vi "Fetch Min Max Waveform.vi"(8 "error in (no error)":errorcluster, 9 "Maximum Time (10000 ms)":u32=10000, 10 "Channel (1: Channel 1)":u16(ring)=1 items=["Channel 1"=1, "Channel 2"=2, "Channel 3"=3, "Channel 4"=4], 11 "VISA resource name":refnum<visa-resource-name>) -> (0 "error out":errorcluster, 1 "Max Waveform Data":waveform(dbl)(graph), 2 "Min Waveform Data":waveform(dbl)(graph), 3 "VISA resource name out":refnum<visa-resource-name>)   [LabVIEW 2011, in "Agilent DSO1000 Series.lvlib"]
doc: "Returns the min and maxwaveform the oscilloscope acquired for the specified channel. This VI only works in Peak Detect acquisiton mode.\n\nYou use the Initiate VI to start an acquisition on the channels that you enable with the Configure Channel VI. The oscilloscope acquires waveforms for the enabled channels concurrently. You must call this VI separately for each enabled channel to obtain the waveforms.\n\nYou can call the Read Waveform VI instead of using low-level VIs.\n\n<B>Note:</B> Use this VI only with other low-level VIs. The high-level VIs automatically incorporate this functionality. This VI does not check the instrument status."
uses:
  <instrlib>/Agilent DSO1000 Series/Agilent DSO1000 Series.lvlib
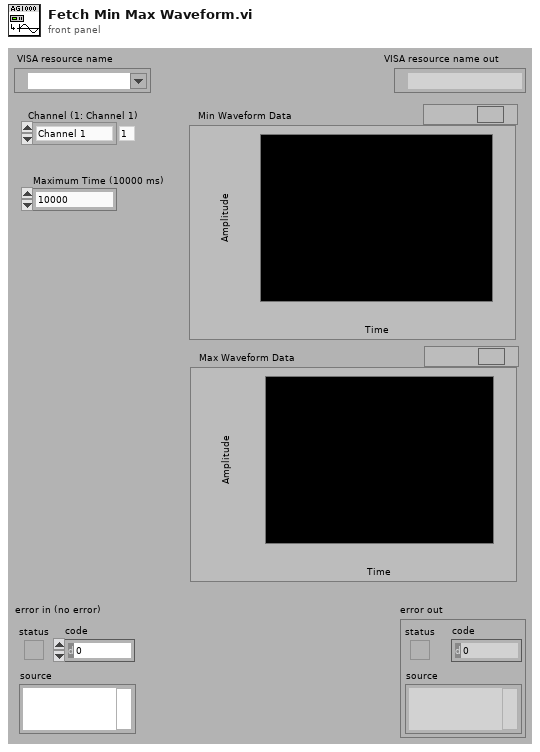
[diagram p1: front panel]
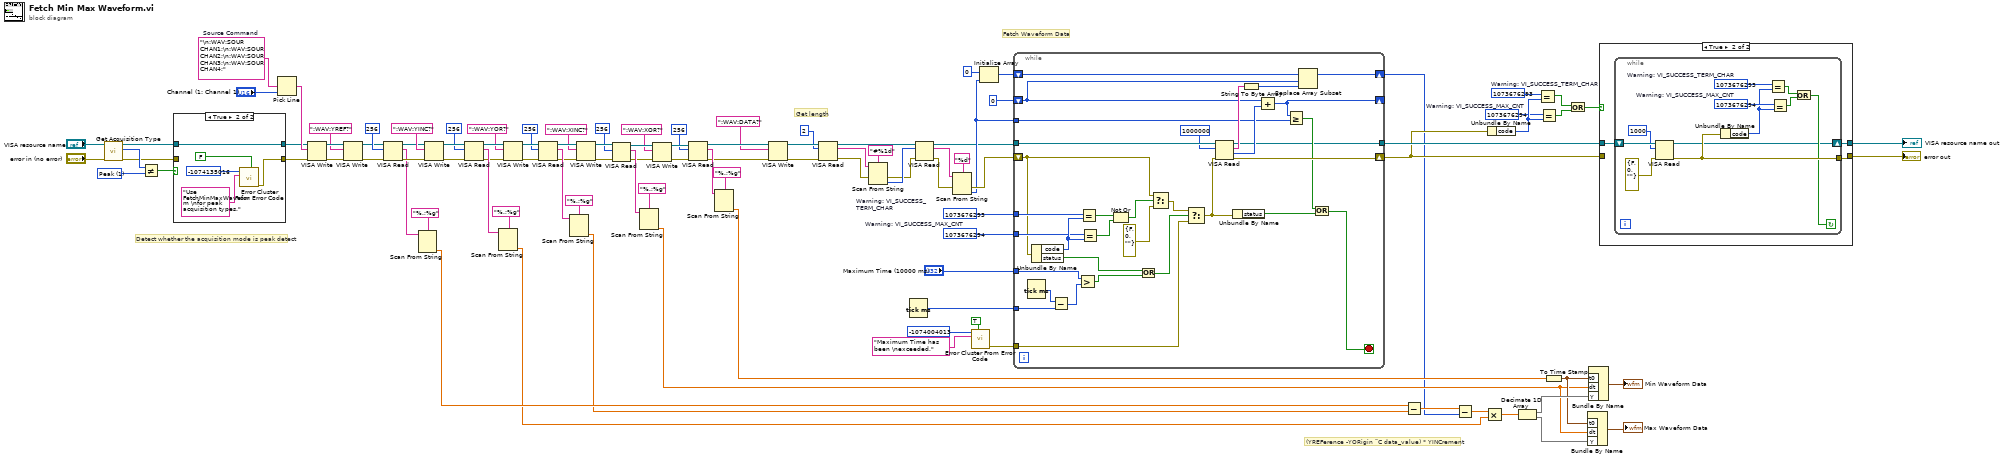
[diagram p0: block diagram]
diagram:
  w29 = 1 items=["Normal", "Peak", "Average"] ("y")
  w35 = 1073676294  # Warning: VI_SUCCESS_MAX_CNT
  w46 = 1073676293  # Warning: VI_SUCCESS_TERM_CHAR
  w51 = 1073676294  # Warning: VI_SUCCESS_MAX_CNT
  w52 = 1073676293  # Warning: VI_SUCCESS_TERM_CHAR
  w103 = "\n:WAV:SOUR CHAN1;\n:WAV:SOUR CHAN2;\n:WAV:SOUR CHAN3;\n:WAV:SOUR CHAN4;"  # Source Command
  # "(YREFerence -YORigin ¨C data_value) * YINCrement"
  # "Detect whether the acquisition mode is peak detect"
  # "Get length"
  # "Fetch Waveform Data"
  n1 = call <instrlib>:"Get Acquisition Type.vi"("error in (no error)"="error in (no error)", "VISA resource name"="VISA resource name") -> ("error out"=w25:errorcluster, "Acquisition Type"=w30:i32, "VISA resource name out"=w27:refnum<visa-resource-name>)  [unwired: 7 in]
  n2 = Not Equal?(x=w30, y=w29) -> (x != y?=w28:bool)
  n3 = case shown="True" w28 {
    tunnel: w27 -> [w107 w112]
    tunnel: [w107 w112] -> w26
    tunnel: w25 -> [w106 _]
    tunnel: [w106 w108] -> w24
    frame False {
    }
    frame True {
      n4 = call <vilib>:"Error Cluster From Error Code.vi"("is warning? (False)"=FALSE, "error message (\"\")"="Use FetchMinMaxWaveform \nfor peak  acquisition types.", "error code (0)"=-1074135016) -> ("error out"=w108:errorcluster)  [unwired: 6 in]
    }
  }
  n5 = Pick Line(multi-line string=w103, line index="Channel (1: Channel 1)") -> (output string=w104:string)  [unwired: 1 in]
  n6 = VISA Write(VISA resource name=w26, write buffer=w104, error in (no error)=w24) -> (VISA resource name out=w20:refnum<visa-resource-name>, error out=w19:errorcluster)  [unwired: 1 out]
  n7 = VISA Write(VISA resource name=w20, write buffer=":WAV:YREF?", error in (no error)=w19) -> (VISA resource name out=w21:refnum<visa-resource-name>, error out=w22:errorcluster)  [unwired: 1 out]
  n8 = VISA Read(VISA resource name=w21, byte count=u32 256, error in (no error)=w22) -> (VISA resource name out=w17:refnum<visa-resource-name>, read buffer=w14:string, error out=w16:errorcluster)  [unwired: 1 out]
  n9 = Scan From String(format string="%.;%g", input string=w14) -> (output 1=w13:dbl)  [unwired: 3 in, 3 out]
  n10 = VISA Write(VISA resource name=w17, write buffer=":WAV:YINC?", error in (no error)=w16) -> (VISA resource name out=w75:refnum<visa-resource-name>, error out=w74:errorcluster)  [unwired: 1 out]
  n11 = VISA Read(VISA resource name=w75, byte count=u32 256, error in (no error)=w74) -> (VISA resource name out=w100:refnum<visa-resource-name>, read buffer=w102:string, error out=w99:errorcluster)  [unwired: 1 out]
  n12 = Scan From String(format string="%.;%g", input string=w102) -> (output 1=w1:dbl)  [unwired: 3 in, 3 out]
  n13 = VISA Write(VISA resource name=w100, write buffer=":WAV:YOR?", error in (no error)=w99) -> (VISA resource name out=w97:refnum<visa-resource-name>, error out=w96:errorcluster)  [unwired: 1 out]
  n14 = VISA Read(VISA resource name=w97, byte count=u32 256, error in (no error)=w96) -> (VISA resource name out=w92:refnum<visa-resource-name>, read buffer=w94:string, error out=w91:errorcluster)  [unwired: 1 out]
  n15 = Scan From String(format string="%.;%g", input string=w94) -> (output 1=w2:dbl)  [unwired: 3 in, 3 out]
  n16 = VISA Write(VISA resource name=w92, write buffer=":WAV:XINC?", error in (no error)=w91) -> (VISA resource name out=w89:refnum<visa-resource-name>, error out=w88:errorcluster)  [unwired: 1 out]
  n17 = VISA Read(VISA resource name=w89, byte count=u32 256, error in (no error)=w88) -> (VISA resource name out=w84:refnum<visa-resource-name>, read buffer=w86:string, error out=w83:errorcluster)  [unwired: 1 out]
  n18 = Scan From String(format string="%.;%g", input string=w86) -> (output 1=w5:dbl)  [unwired: 3 in, 3 out]
  n19 = VISA Write(VISA resource name=w84, write buffer=":WAV:XOR?", error in (no error)=w83) -> (VISA resource name out=w81:refnum<visa-resource-name>, error out=w80:errorcluster)  [unwired: 1 out]
  n20 = VISA Read(VISA resource name=w81, byte count=u32 256, error in (no error)=w80) -> (VISA resource name out=w37:refnum<visa-resource-name>, read buffer=w78:string, error out=w36:errorcluster)  [unwired: 1 out]
  n21 = Scan From String(format string="%.;%g", input string=w78) -> (output 1=w72:dbl)  [unwired: 3 in, 3 out]
  n22 = VISA Write(VISA resource name=w37, write buffer=":WAV:DATA?" ("multi-line string"), error in (no error)=w36) -> (VISA resource name out=w71:refnum<visa-resource-name>, error out=w70:errorcluster)  [unwired: 1 out]
  n23 = VISA Read(VISA resource name=w71, byte count=u32 2, error in (no error)=w70) -> (VISA resource name out=w66:refnum<visa-resource-name>, read buffer=w67:string, error out=w68:errorcluster)  [unwired: 1 out]
  n24 = Scan From String(format string="#%1d", input string=w67, error in=w68) -> (error out=w63:errorcluster, output 1=w64:i32)  [unwired: 2 in, 2 out]
  n25 = Tick Count (ms)() -> (millisecond timer value=w53:u32)
  n26 = VISA Read(VISA resource name=w66, byte count=w64, error in (no error)=w63) -> (VISA resource name out=w54:refnum<visa-resource-name>, read buffer=w61:string, error out=w62:errorcluster)  [unwired: 1 out]
  n27 = Scan From String(format string="%d", input string=w61, error in=w62) -> (error out=w59:errorcluster, output 1=w55:i32)  [unwired: 2 in, 2 out]
  n28 = call <vilib>:"Error Cluster From Error Code.vi"("show call chain? (False)"=TRUE, "error message (\"\")"="Maximum Time has been \nexceeded." ("error message (\"\")"), "error code (0)"=-1074004013) -> ("error out"=w47:errorcluster)  [unwired: 6 in]
  n29 = Initialize Array(i8 0 ("element"), w55) -> (w57:i8[])
  n30 = while {
    shift-right: [w115] -> w3
    shift-left: w57 -> [w116]
    shift-right: [w123] -> _
    shift-left: 0 ("element") -> [w117]
    tunnel: w55 -> [w122]
    tunnel: w54 -> [w142]
    shift-right: [w126] -> w40
    shift-left: w59 -> [w136]
    tunnel: w53 -> [w145]
    tunnel: w52 -> [w140]
    tunnel: w51 -> [w139]
    tunnel: w47 -> [w129]
    tunnel: [w114] -> w41
    tunnel: "Maximum Time (10000 ms)" -> [w113]
    stop <- w119 stop-if-true
    n31 = Tick Count (ms)() -> (millisecond timer value=w144:u32)
    n32 = Unbundle By Name(w136) -> ("code"=w141:i32, "status"=w132:bool)
    n33 = Subtract(x=w144, y=w145) -> (x-y=w143:u32)
    n34 = Greater?(x=w113, y=w143) -> (0:w133:bool)
    n35 = Equal?(x=w140, y=w141) -> (x = y?=w138:bool)
    n36 = Equal?(x=w139, y=w141) -> (x = y?=w137:bool)
    n37 = Not Or(1:w137, 2:w138) -> (0:w135:bool)
    n38 = Or(x=w132, y=w133) -> (x .or. y?=w131:bool)
    n39 = Select(t=w136, s=w135, f=errorcluster {"status"=FALSE, "code"=0, "source"=""} ("error in (no error) 2")) -> (s? t:f=w130:errorcluster)
    n40 = Select(t=w130, s=w131, f=w129) -> (s? t:f=w128:errorcluster)
    n41 = VISA Read(VISA resource name=w142, byte count=u32 1000000, error in (no error)=w128) -> (VISA resource name out=w114:refnum<visa-resource-name>, read buffer=w125:string, return count=w124:u32, error out=w126:errorcluster)
    n42 = Unbundle By Name(w128) -> ("status"=w120:bool)
    n43 = String To Byte Array(string=w125) -> (unsigned byte array=w118:u8[])
    n44 = Add(x=w117, y=w124) -> (x+y=w123:u32)
    n45 = Greater Or Equal?(x=w123, y=w122) -> (x >= y?=w121:bool)
    n46 = Replace Array Subset(array=w116, new element=w118, index=w117) -> (w115:i8[])
    n47 = Or(x=w121, y=w120) -> (x .or. y?=w119:bool)
  }
  n48 = Subtract(x=w13, y=w2) -> (x-y=w12:dbl)
  n49 = Subtract(x=w12, y=w3) -> (x-y=w11:dbl[])
  n50 = Multiply(x=w11, y=w1) -> (x*y=w10:dbl[])
  n51 = Unbundle By Name(w40) -> ("code"=w45:i32)
  n52 = Decimate 1D Array(w10) -> (w8:dbl[], w7:dbl[])
  n53 = Equal?(x=w46, y=w45) -> (x = y?=w44:bool)
  n54 = Equal?(x=w35, y=w45) -> (x = y?=w43:bool)
  n55 = To Time Stamp(1:w72) -> (0:w6:timestamp)
  n56 = Or(x=w44, y=w43) -> (x .or. y?=w42:bool)
  n57 = Bundle By Name("t0"=w6, "dt"=w5, "Y"=w7) -> (→"Max Waveform Data":waveform(dbl))  [unwired: 1 in]
  n58 = Bundle By Name("t0"=w6, "dt"=w5, "Y"=w8) -> (→"Min Waveform Data":waveform(dbl))  [unwired: 1 in]
  n59 = case shown="True" w42 {
    tunnel: w41 -> [w147 w150]
    tunnel: w40 -> [w146 _]
    tunnel: [w147 w148] -> w39
    tunnel: [w146 w149] -> w38
    frame False {
    }
    frame True {
      n60 = while {
        shift-right: [w151] -> w148
        shift-left: w150 -> [w161]
        tunnel: [w154] -> w149
        stop <- w152 continue-if-true
        w157 = 1073676294  # Warning: VI_SUCCESS_MAX_CNT
        w158 = 1073676293  # Warning: VI_SUCCESS_TERM_CHAR
        n61 = VISA Read(VISA resource name=w161, byte count=u32 1000, error in (no error)=errorcluster {"status"=FALSE, "code"=0, "source"=""} ("error in (no error) 2")) -> (VISA resource name out=w151:refnum<visa-resource-name>, error out=w154:errorcluster)  [unwired: 2 out]
        n62 = Unbundle By Name(w154) -> ("code"=w153:i32)
        n63 = Equal?(x=w158, y=w153) -> (x = y?=w156:bool)
        n64 = Equal?(x=w157, y=w153) -> (x = y?=w155:bool)
        n65 = Or(x=w156, y=w155) -> (x .or. y?=w152:bool)
      }
    }
  }
  "error out" <- w38
  "VISA resource name out" <- w39
